vi "Camera_Config_Specific_Attributes_2.0.vi"(4 "Crop?":bool, 5 "Camera":T5, 6 "Detect Movement":bool, 8 "error in (no error)":errorcluster, 10 "Refnum in":T2, 11 "Data":T1={"Camera 1"={"Camera1"="", "Cam 1"=FALSE, "CAM1 Model"=enum."a2A5328-15ucBAS", "Cam1 ID"=0}, "Camera 2"={"Camera2"="", "Cam 2"=FALSE, "CAM2 Model"=enum."a2A5328-15ucBAS", "Cam2 ID"=0}, "Image"={"Camera1_Img"=refnum, "Camera2_Img"=refnum, "Img1_Orig_Disp"=refnum, "Img2_Orig_Disp"=refnum, "Img1_Orig_RGB"=refnum, "Img2_Orig_RGB"=refnum, "Blue_Plane_Extract"=refnum, "Subtracted_Plane"=refnum, "Img1_Binary"=refnum, "Img2_Binary"=refnum, "Crop_Mask"=refnum, "Img1_Save"=refnum, "Img2_Save"=refnum, "Img1_Cali_Full"=refnum, "Img2_Cali_Full"=refnum, "Img1_Cali_Detect"=refnum, "Img2_Cali_Detect"=refnum}, "Ques"={"Cam 1 queue"=refnum, "Cam 2 queue"=refnum, "Cam 1 - save queue"=refnum, "Cam 2 - save queue"=refnum, "Image Process Queue Size"=500, "Image Save Queue Size"=500, "Overload threshold"=500, "Max large object threshold"=0}, "Arduino SRS"={"Pinch-valve"="", "Actuator"=FALSE, "Arduino Uno"="", "Valve state"=enum."Open"}, "Pump"={"Port"="", "Connection"=FALSE, "Flush Size"=0, "Command"="", "Pump Size"=enum."None", "Pump"="", "Ready"=FALSE}, "Camera settings"={"Detection settings"={"Sample size threshold"=500, "Detection Region %"=30.0, "Timeout Sample"=200}, "Lens/camera settings"={"Aperture"=enum."Item 0", "Legacy Cam Attributes"=FALSE, "Max Framerate"=100, "Exposure Time"=1000.0, "Framerate"=15}, "Crop settings"={"Cam1"={"Rectangle 1"={"Left"=0, "Top"=0, "Right"=0, "Bottom"=0, "Rotation"=0.0}, "Camera Orientation 1"="", "Pixel to mm 1"=0.0}, "Cam2"={"Rectangle 2"={"Left"=0, "Top"=0, "Right"=0, "Bottom"=0, "Rotation"=0.0}, "Camera Orientation 2"="", "Pixel to mm 2"=0.0}}}, "Arduino ISS"={"Mega F3"="", "Phase3"=FALSE, "Barcode"="", "Sorting sys."=FALSE, "Initial size"=0.0, "Size Interval"=0.0, "Mun. of containers"=0.0, "Container nr."=0.0, "Arduino Mega"=""}, "Img_Capt"=FALSE, "Empty_Refill"=FALSE, "I don't think is in use"={"Light intensity"=100}, "Extended setup"={"Location"="Station", "Latitude"="Station", "Longitude"="Station", "Determiner"="Station", "Sex"="Station", "Station"="", "Collection date"=""}, "Main interface"={"Sample Name"="Test Sample", "Operator"="JFR", "Species Name"="", "Other Notes"=""}, "Tap1"=0, "SystemVersion"=0, "System Serial"="", "Exit"=FALSE, "Kuvette Full"=FALSE, "Core JKI"={"Current VI Reference"=refnum, "Close Panel on Exit?"=FALSE}, "Calibration"={"Calibration 1"=path "C:/Users/au540322/Desktop/IHS_Project/images/Debris/Debris_0/Debris_0_2019_06_01-23-32-49-686.PNG", "Calibration 2"=path "C:/Users/au540322/Desktop/IHS_Project/images/Debris/Debris_0/Debris_0_2019_06_01-23-32-49-686.PNG", "Detect 1"=path "C:/Users/au540322/Desktop/IHS_Project/images/Debris/Debris_0/Debris_0_2019_06_01-23-32-49-686.PNG", "Detect 2"=path "C:/Users/au540322/Desktop/IHS_Project/images/Debris/Debris_0/Debris_0_2019_06_01-23-32-49-686.PNG"}, "Auto Flush"=FALSE, "Status History"="", "Timestamp Start"=""} {"SystemVersion" items=["Standard", "XL"]; "Tap1" items=["Session Data", "Extended Setup", "Buffer", "Camera", "Dispenser", "Stats", "Connections"]; "I don't think is in use"."Light intensity" scale=0.0..100.0; "Camera settings"."Crop settings"."Cam2"."Rectangle 2"."Rotation" format="%.2f"; "Camera settings"."Crop settings"."Cam2"."Rectangle 2"."Left" scale=0.0..1024.0; "Camera settings"."Crop settings"."Cam2"."Rectangle 2"."Right" scale=0.0..1024.0; "Camera settings"."Crop settings"."Cam1"."Rectangle 1"."Rotation" format="%.2f"; "Camera settings"."Crop settings"."Cam1"."Rectangle 1"."Left" scale=0.0..1024.0; "Camera settings"."Crop settings"."Cam1"."Rectangle 1"."Right" scale=0.0..1024.0; "Camera settings"."Lens/camera settings"."Framerate" min=1; "Camera settings"."Lens/camera settings"."Max Framerate" min=1; "Camera settings"."Detection settings"."Sample size threshold" min=1; "Pump"."Flush Size" min=0 max=6000 step=100; "Ques"."Overload threshold" min=1; "Ques"."Image Save Queue Size" min=1; "Ques"."Image Process Queue Size" min=1}) -> (0 "error out":errorcluster, 3 "Refnum out":T2)   [LabVIEW 2024]
uses:
  <vilib>/userDefined/High Color/IMAQdx.ctl
  Camera_ID.ctl
  controls/Data_JKI.ctl
  <vilib>/vision/Image Controls.llb/IMAQ Image.ctl
  <resource>/objmgr/imaqdx.rc
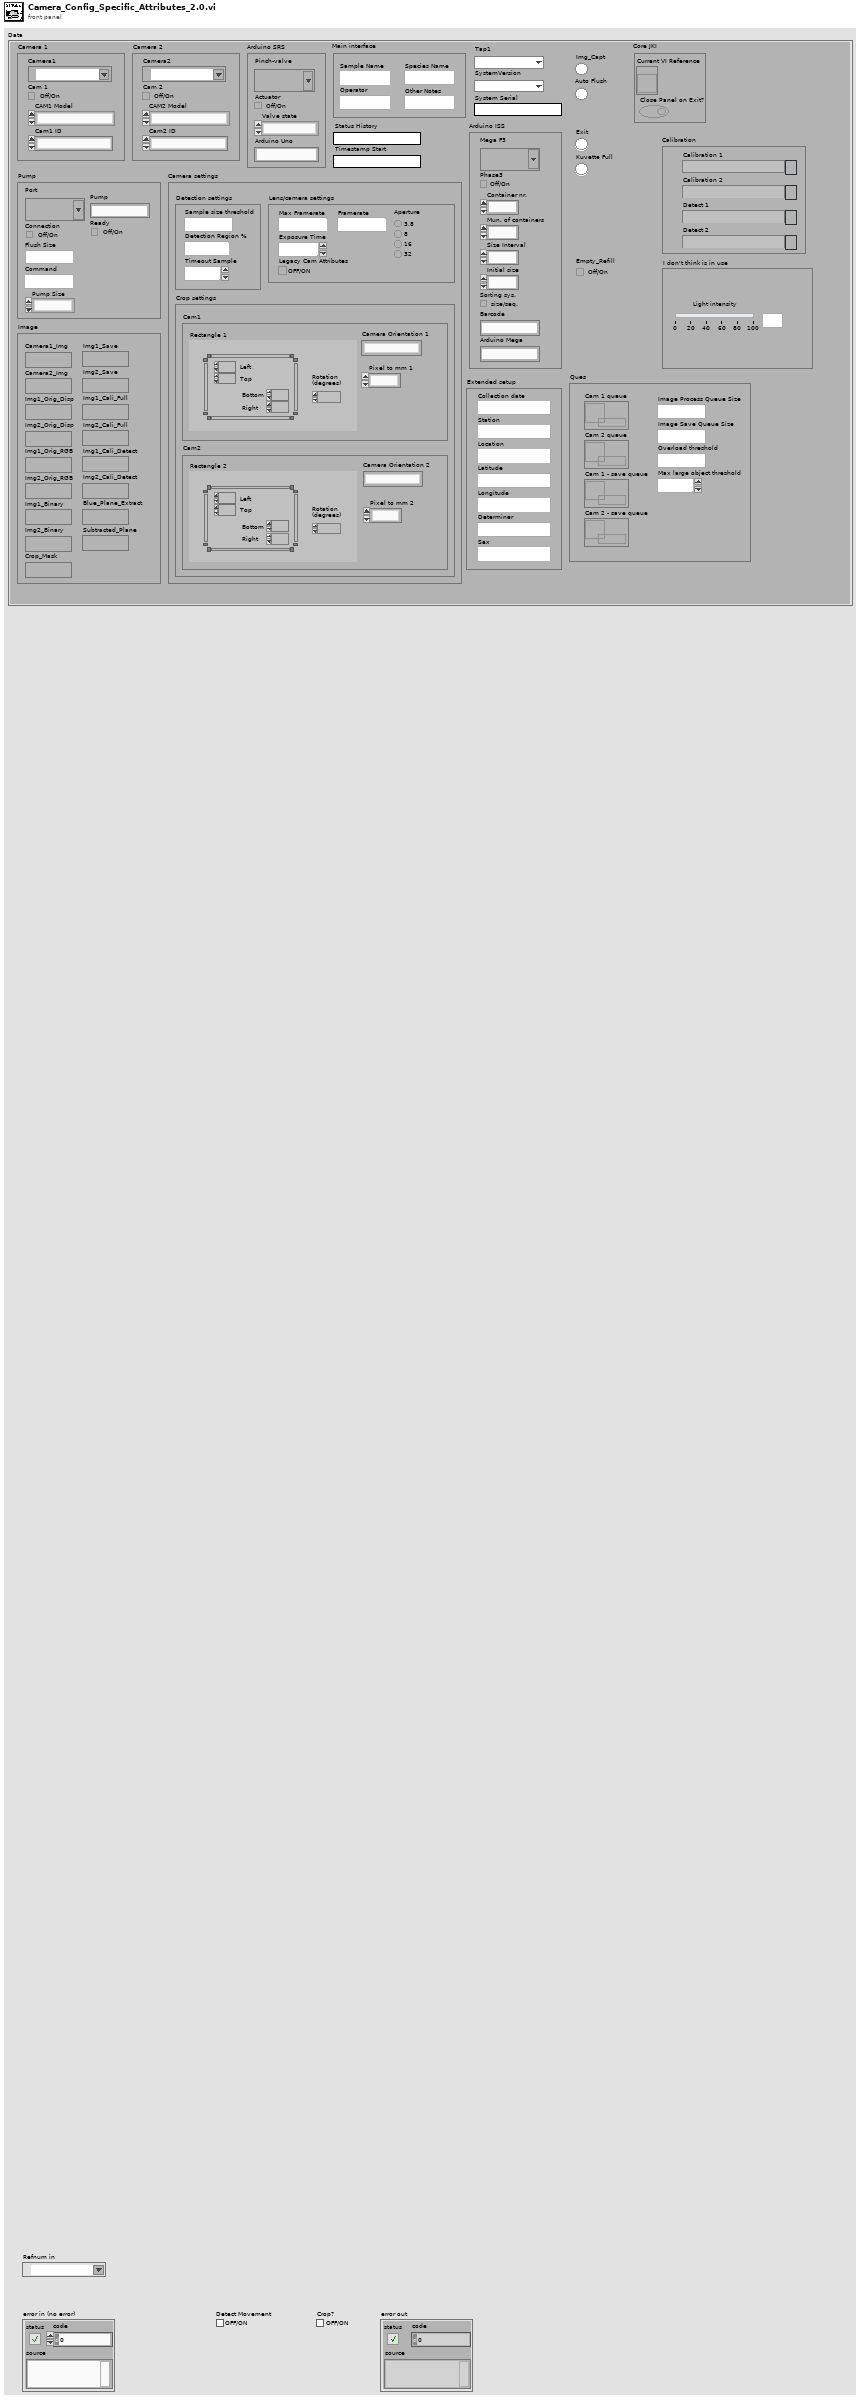
[diagram p1: front panel]
types:
  T1 = typedef "Data_JKI.ctl" = cluster{"Camera 1":cluster{"Camera1":T2, "Cam 1":bool, "CAM1 Model":enum16{"a2A5328-15ucBAS", "acA1920-155uc"}, "Cam1 ID":i32}, "Camera 2":cluster{"Camera2":T2, "Cam 2":bool, "CAM2 Model":enum16{"a2A5328-15ucBAS", "acA1920-155uc"}, "Cam2 ID":i32}, "Image":cluster{"Camera1_Img":T3, "Camera2_Img":T3, "Img1_Orig_Disp":T3, "Img2_Orig_Disp":T3, "Img1_Orig_RGB":T3, "Img2_Orig_RGB":T3, "Blue_Plane_Extract":T3, "Subtracted_Plane":T3, "Img1_Binary":T3, "Img2_Binary":T3, "Crop_Mask":T3, "Img1_Save":T3, "Img2_Save":T3, "Img1_Cali_Full":T3, "Img2_Cali_Full":T3, "Img1_Cali_Detect":T3, "Img2_Cali_Detect":T3}, "Ques":cluster{"Cam 1 queue":refnum<queue>, "Cam 2 queue":refnum<queue>, "Cam 1 - save queue":refnum<queue>, "Cam 2 - save queue":refnum<queue>, "Image Process Queue Size":i32, "Image Save Queue Size":i32, "Overload threshold":i32, "Max large object threshold":i32}, "Arduino SRS":cluster{"Pinch-valve":refnum<visa-resource-name>, "Actuator":bool, "Arduino Uno":string, "Valve state":enum16{"Standby", "Close", "Open"}}, "Pump":cluster{"Port":refnum<visa-resource-name>, "Connection":bool, "Flush Size":i32, "Command":string, "Pump Size":enum16{"None", "Small", "Large"}, "Pump":string, "Ready":bool}, "Camera settings":cluster{"Detection settings":cluster{"Sample size threshold":i32, "Detection Region %":dbl, "Timeout Sample":i32}, "Lens/camera settings":cluster{"Aperture":enum32{"Item 0", "Item 1", "Item 2", "Item 3"}, "Legacy Cam Attributes":bool, "Max Framerate":i32, "Exposure Time":dbl, "Framerate":i32}, "Crop settings":cluster{"Cam1":cluster{"Rectangle 1":T4, "Camera Orientation 1":string, "Pixel to mm 1":dbl}, "Cam2":cluster{"Rectangle 2":T4, "Camera Orientation 2":string, "Pixel to mm 2":dbl}}}, "Arduino ISS":cluster{"Mega F3":refnum<visa-resource-name>, "Phase3":bool, "Barcode":string, "Sorting sys.":bool, "Initial size":dbl, "Size Interval":dbl, "Mun. of containers":dbl, "Container nr.":dbl, "Arduino Mega":string}, "Img_Capt":bool, "Empty_Refill":bool, "I don't think is in use":cluster{"Light intensity":i32}, "Extended setup":cluster{"Location":string, "Latitude":string, "Longitude":string, "Determiner":string, "Sex":string, "Station":string, "Collection date":string}, "Main interface":cluster{"Sample Name":string, "Operator":string, "Species Name":string, "Other Notes":string}, "Tap1":u16, "SystemVersion":u16, "System Serial":string, "Exit":bool, "Kuvette Full":bool, "Core JKI":cluster{"Current VI Reference":refnum<vi>, "Close Panel on Exit?":bool}, "Calibration":cluster{"Calibration 1":path, "Calibration 2":path, "Detect 1":path, "Detect 2":path}, "Auto Flush":bool, "Status History":string, "Timestamp Start":string}
  T2 = typedef "IMAQdx.ctl" = refnum<k21>
  T3 = typedef "IMAQ Image.ctl" = refnum<image>
  T4 = typedef "IMAQ Rectangle" = cluster{"Left":i32, "Top":i32, "Right":i32, "Bottom":i32, "Rotation":dbl}
  T5 = typedef "Camera_ID.ctl" = enum16{"Camera 1", "Camera 2"}
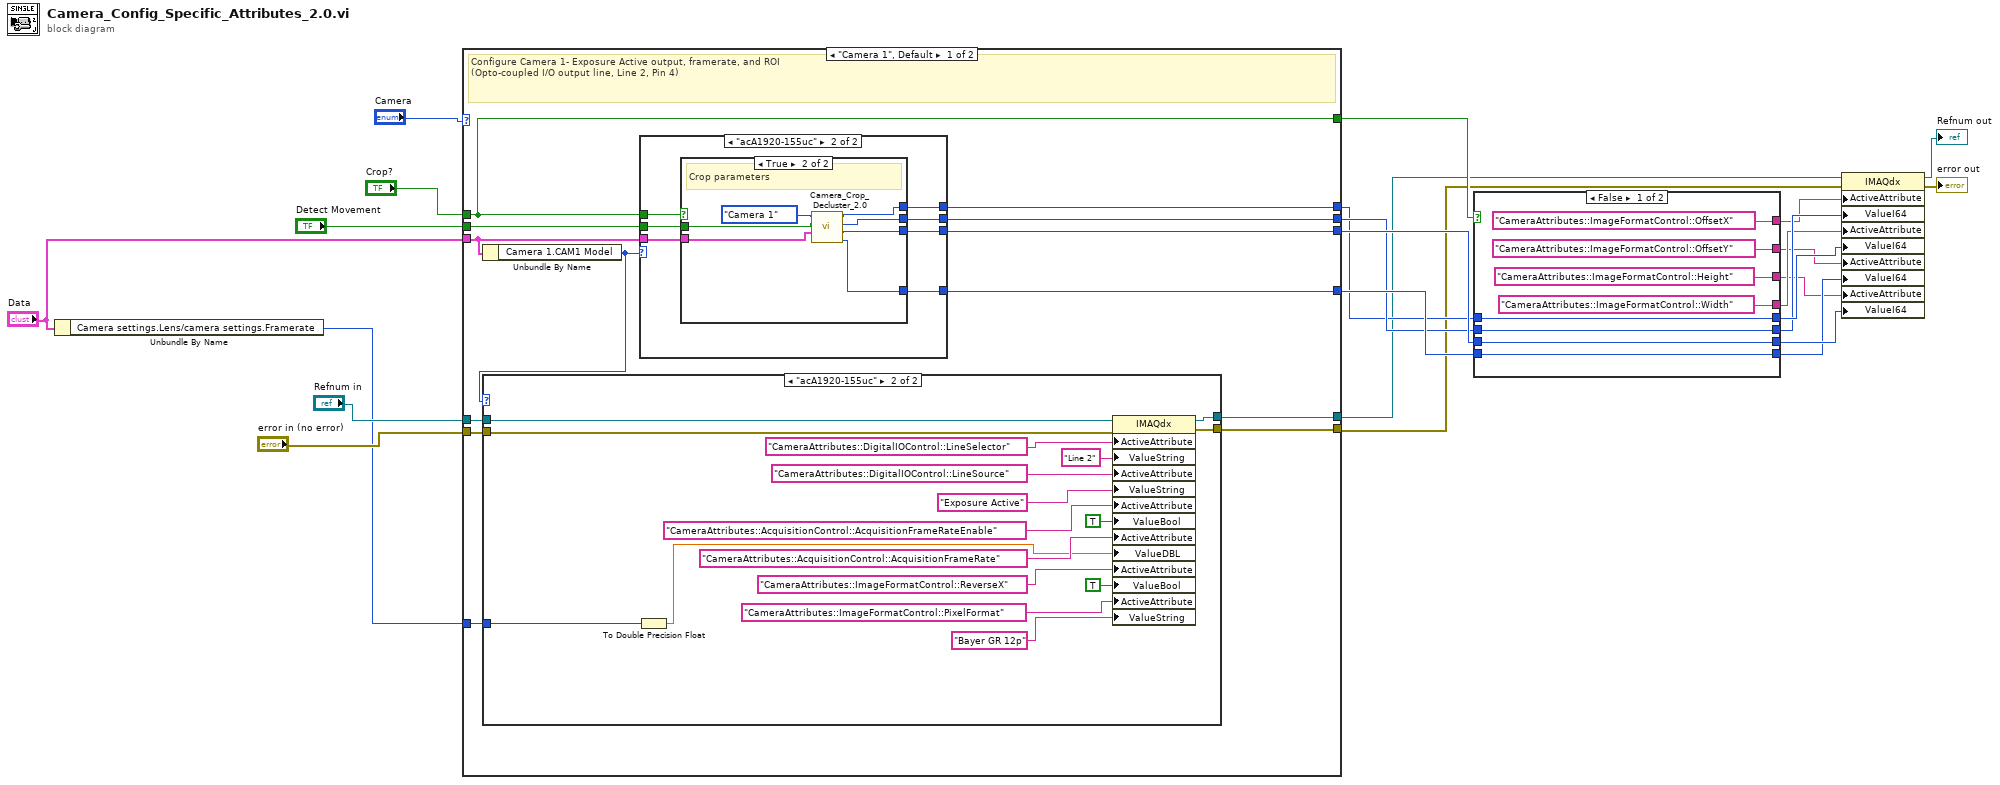
[diagram p0: block diagram]
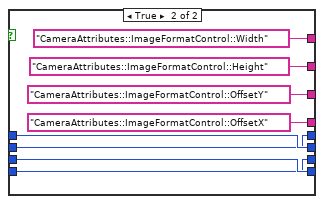
[diagram p2: hidden frame]
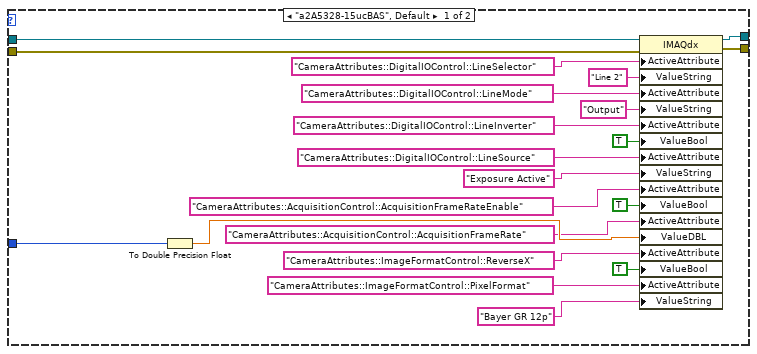
[diagram p3: hidden frame]
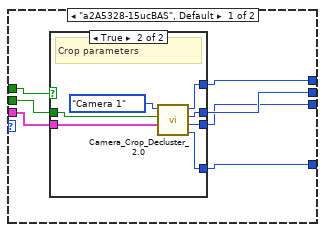
[diagram p4: hidden frame]
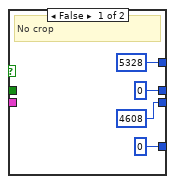
[diagram p5: hidden frame]
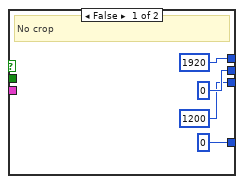
[diagram p6: hidden frame]
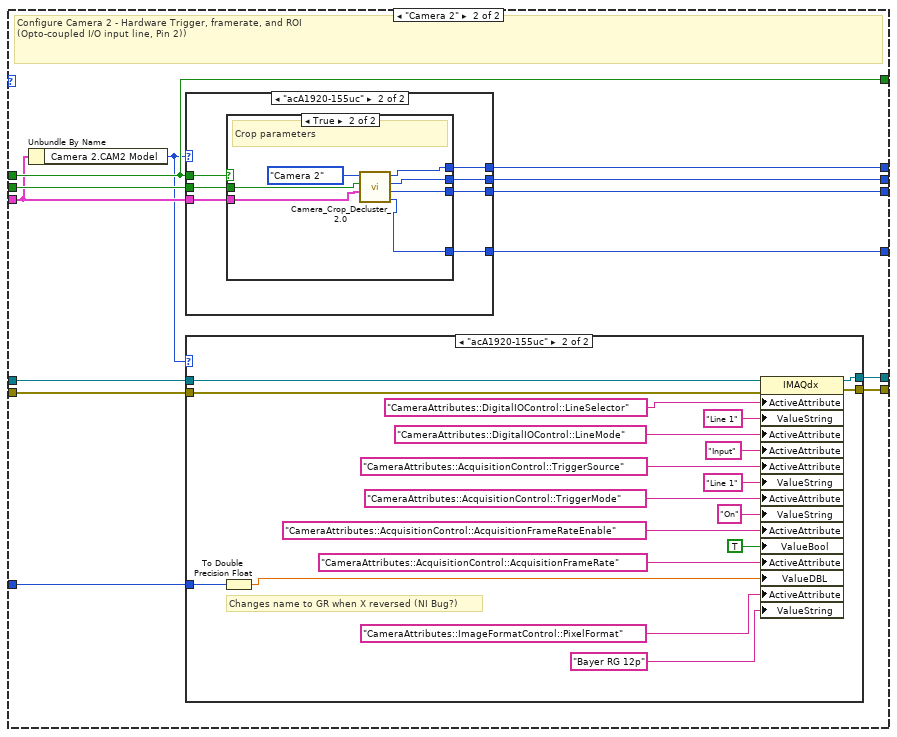
[diagram p7: hidden frame]
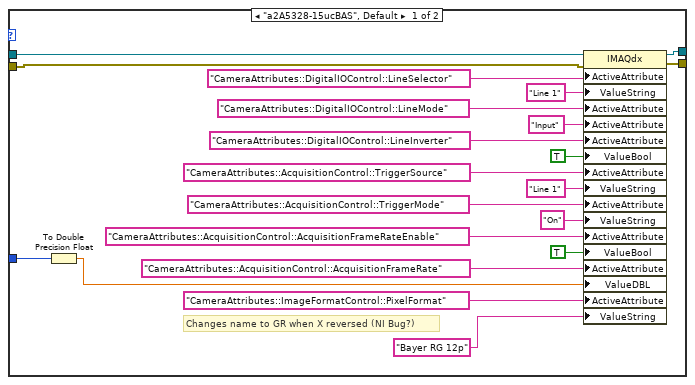
[diagram p8: hidden frame]
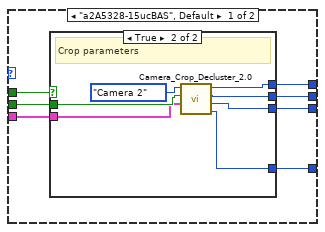
[diagram p9: hidden frame]
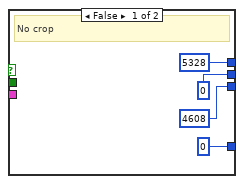
[diagram p10: hidden frame]
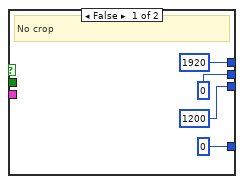
[diagram p11: hidden frame]
diagram:
  n1 = Unbundle By Name("Data") -> ("Camera settings.Lens/camera settings.Framerate"=w4:i32)
  n2 = case shown="\"Camera 1\", Default" "Camera" {
    tunnel: "Refnum in" -> [w37 w118]
    tunnel: [w36 w117] -> w2
    tunnel: [w35 w116] -> w1
    tunnel: w4 -> [w27 w113]
    tunnel: [w33 w124] -> w17
    tunnel: [w34 w123] -> w14
    tunnel: [w31 w121] -> w19
    tunnel: [w32 w122] -> w15
    tunnel: "Crop?" -> [w30 w120]
    tunnel: [w30 w120] -> w12
    tunnel: "Data" -> [w26 w114]
    tunnel: "Detect Movement" -> [w29 w119]
    tunnel: "error in (no error)" -> [w28 w115]
    frame "Camera 1", Default {
      # "Configure Camera 1- Exposure Active output, framerate, and ROI\n(Opto-coupled I/O output line, Line 2, Pin 4)"
      n3 = Unbundle By Name(w26) -> ("Camera 1.CAM1 Model"=w25:enum16{"a2A5328-15ucBAS", "acA1920-155uc"})
      n4 = case shown="\"acA1920-155uc\"" w25 {
        tunnel: w37 -> [w58 w75]
        tunnel: [w56 w74] -> w36
        tunnel: [w55 w73] -> w35
        tunnel: w28 -> [w57 w71]
        tunnel: w27 -> [w44 w60]
        frame "a2A5328-15ucBAS", Default {
          n5 = To Double Precision Float(number=w44) -> (double precision float=w43:dbl)
          n6 = property class="IMAQdx"(reference=w58, error in=w57, "ActiveAttribute"="CameraAttributes::DigitalIOControl::LineSelector", "ValueString"="Line 2", "ActiveAttribute"="CameraAttributes::DigitalIOControl::LineMode", "ValueString"="Output", "ActiveAttribute"="CameraAttributes::DigitalIOControl::LineInverter", "ValueBool"=TRUE, "ActiveAttribute"="CameraAttributes::DigitalIOControl::LineSource", "ValueString"="Exposure Active", "ActiveAttribute"="CameraAttributes::AcquisitionControl::AcquisitionFrameRateEnable", "ValueBool"=TRUE, "ActiveAttribute"="CameraAttributes::AcquisitionControl::AcquisitionFrameRate", "ValueDBL"=w43, "ActiveAttribute"="CameraAttributes::ImageFormatControl::ReverseX", "ValueBool"=TRUE, "ActiveAttribute"="CameraAttributes::ImageFormatControl::PixelFormat", "ValueString"="Bayer GR 12p") -> (reference out=w56:T2, error out=w55:errorcluster)
        }
        frame "acA1920-155uc" {
          n7 = To Double Precision Float(number=w60) -> (double precision float=w59:dbl)
          n8 = property class="IMAQdx"(reference=w75, error in=w71, "ActiveAttribute"="CameraAttributes::DigitalIOControl::LineSelector", "ValueString"="Line 2", "ActiveAttribute"="CameraAttributes::DigitalIOControl::LineSource", "ValueString"="Exposure Active", "ActiveAttribute"="CameraAttributes::AcquisitionControl::AcquisitionFrameRateEnable", "ValueBool"=TRUE, "ActiveAttribute"="CameraAttributes::AcquisitionControl::AcquisitionFrameRate", "ValueDBL"=w59, "ActiveAttribute"="CameraAttributes::ImageFormatControl::ReverseX", "ValueBool"=TRUE, "ActiveAttribute"="CameraAttributes::ImageFormatControl::PixelFormat", "ValueString"="Bayer GR 12p") -> (reference out=w74:T2, error out=w73:errorcluster)
        }
      }
      n9 = case shown="\"acA1920-155uc\"" w25 {
        tunnel: [w79 w100] -> w34
        tunnel: [w77 w99] -> w33
        tunnel: [w78 w98] -> w32
        tunnel: [w76 w97] -> w31
        tunnel: w30 -> [w82 w96]
        tunnel: w26 -> [w80 w95]
        tunnel: w29 -> [w81 w94]
        frame "a2A5328-15ucBAS", Default {
          n10 = case shown="True" w82 {
            tunnel: [5328 w90] -> w79
            tunnel: [4608 w88] -> w77
            tunnel: [i64 0 w89] -> w78
            tunnel: [0 w87] -> w76
            tunnel: w80 -> [_ w91]
            tunnel: w81 -> [_ w92]
            frame False {
              # "No crop"
            }
            frame True {
              # "Crop parameters"
              n11 = call "Camera_Crop_Decluster_2.0.vi"("Data"=w91, "Detect Movement"=w92, "Camera"=Camera_ID."Camera 1") -> ("OffsetY"=w87:i64, "Height"=w88:i64, "OffsetX"=w89:i64, "Width"=w90:i64)  [unwired: 5 in]
            }
          }
        }
        frame "acA1920-155uc" {
          n12 = case shown="True" w96 {
            tunnel: [i64 1920 w108] -> w100
            tunnel: [1200 w106] -> w99
            tunnel: [i64 0 w107] -> w98
            tunnel: [0 w105] -> w97
            tunnel: w95 -> [_ w109]
            tunnel: w94 -> [_ w110]
            frame False {
              # "No crop"
            }
            frame True {
              # "Crop parameters"
              n13 = call "Camera_Crop_Decluster_2.0.vi"("Data"=w109, "Detect Movement"=w110, "Camera"=Camera_ID."Camera 1") -> ("OffsetY"=w105:i64, "Height"=w106:i64, "OffsetX"=w107:i64, "Width"=w108:i64)  [unwired: 5 in]
            }
          }
        }
      }
    }
    frame "Camera 2" {
      # "Configure Camera 2 - Hardware Trigger, framerate, and ROI \n(Opto-coupled I/O input line, Pin 2))"
      n14 = Unbundle By Name(w114) -> ("Camera 2.CAM2 Model"=w112:enum16{"a2A5328-15ucBAS", "acA1920-155uc"})
      n15 = case shown="\"acA1920-155uc\"" w112 {
        tunnel: [w166 w189] -> w124
        tunnel: [w168 w188] -> w123
        tunnel: [w167 w187] -> w122
        tunnel: [w165 w186] -> w121
        tunnel: w120 -> [w171 w185]
        tunnel: w114 -> [w170 w184]
        tunnel: w119 -> [w169 w183]
        frame "a2A5328-15ucBAS", Default {
          n16 = case shown="True" w171 {
            tunnel: [i64 4608 w177] -> w166
            tunnel: [i64 5328 w179] -> w168
            tunnel: [i64 0 w178] -> w167
            tunnel: [i64 0 w176] -> w165
            tunnel: w170 -> [_ w180]
            tunnel: w169 -> [_ w181]
            frame False {
              # "No crop"
            }
            frame True {
              # "Crop parameters"
              n17 = call "Camera_Crop_Decluster_2.0.vi"("Data"=w180, "Detect Movement"=w181, "Camera"=Camera_ID."Camera 2") -> ("OffsetY"=w176:i64, "Height"=w177:i64, "OffsetX"=w178:i64, "Width"=w179:i64)  [unwired: 5 in]
            }
          }
        }
        frame "acA1920-155uc" {
          n18 = case shown="True" w185 {
            tunnel: [i64 1200 w195] -> w189
            tunnel: [i64 1920 w197] -> w188
            tunnel: [i64 0 w196] -> w187
            tunnel: [i64 0 w194] -> w186
            tunnel: w184 -> [_ w198]
            tunnel: w183 -> [_ w199]
            frame False {
              # "No crop"
            }
            frame True {
              # "Crop parameters"
              n19 = call "Camera_Crop_Decluster_2.0.vi"("Data"=w198, "Detect Movement"=w199, "Camera"=Camera_ID."Camera 2") -> ("OffsetY"=w194:i64, "Height"=w195:i64, "OffsetX"=w196:i64, "Width"=w197:i64)  [unwired: 5 in]
            }
          }
        }
      }
      n20 = case shown="\"acA1920-155uc\"" w112 {
        tunnel: w118 -> [w129 w163]
        tunnel: [w131 w162] -> w117
        tunnel: [w130 w161] -> w116
        tunnel: w115 -> [w128 w160]
        tunnel: w113 -> [w125 w155]
        frame "a2A5328-15ucBAS", Default {
          # "Changes name to GR when X reversed (NI Bug?)"
          n21 = To Double Precision Float(number=w125) -> (double precision float=w140:dbl)
          n22 = property class="IMAQdx"(reference=w129, error in=w128, "ActiveAttribute"="CameraAttributes::DigitalIOControl::LineSelector", "ValueString"="Line 1", "ActiveAttribute"="CameraAttributes::DigitalIOControl::LineMode", "ActiveAttribute"="Input", "ActiveAttribute"="CameraAttributes::DigitalIOControl::LineInverter", "ValueBool"=TRUE, "ActiveAttribute"="CameraAttributes::AcquisitionControl::TriggerSource", "ValueString"="Line 1", "ActiveAttribute"="CameraAttributes::AcquisitionControl::TriggerMode", "ValueString"="On", "ActiveAttribute"="CameraAttributes::AcquisitionControl::AcquisitionFrameRateEnable", "ValueBool"=TRUE, "ActiveAttribute"="CameraAttributes::AcquisitionControl::AcquisitionFrameRate", "ValueDBL"=w140, "ActiveAttribute"="CameraAttributes::ImageFormatControl::PixelFormat", "ValueString"="Bayer RG 12p") -> (reference out=w131:T2, error out=w130:errorcluster)
        }
        frame "acA1920-155uc" {
          # "Changes name to GR when X reversed (NI Bug?)"
          n23 = To Double Precision Float(number=w155) -> (double precision float=w154:dbl)
          n24 = property class="IMAQdx"(reference=w163, error in=w160, "ActiveAttribute"="CameraAttributes::DigitalIOControl::LineSelector", "ValueString"="Line 1", "ActiveAttribute"="CameraAttributes::DigitalIOControl::LineMode", "ActiveAttribute"="Input", "ActiveAttribute"="CameraAttributes::AcquisitionControl::TriggerSource", "ValueString"="Line 1", "ActiveAttribute"="CameraAttributes::AcquisitionControl::TriggerMode", "ValueString"="On", "ActiveAttribute"="CameraAttributes::AcquisitionControl::AcquisitionFrameRateEnable", "ValueBool"=TRUE, "ActiveAttribute"="CameraAttributes::AcquisitionControl::AcquisitionFrameRate", "ValueDBL"=w154, "ActiveAttribute"="CameraAttributes::ImageFormatControl::PixelFormat", "ValueString"="Bayer RG 12p") -> (reference out=w162:T2, error out=w161:errorcluster)
        }
      }
    }
  }
  n25 = case shown="False" w12 {
    tunnel: ["CameraAttributes::ImageFormatControl::Height" ("ActiveAttribute") "CameraAttributes::ImageFormatControl::OffsetY" ("ActiveAttribute")] -> w6
    tunnel: ["CameraAttributes::ImageFormatControl::OffsetY" ("ActiveAttribute") "CameraAttributes::ImageFormatControl::Height" ("ActiveAttribute")] -> w7
    tunnel: ["CameraAttributes::ImageFormatControl::Width" ("ActiveAttribute") "CameraAttributes::ImageFormatControl::OffsetX" ("ActiveAttribute")] -> w8
    tunnel: ["CameraAttributes::ImageFormatControl::OffsetX" ("ActiveAttribute") "CameraAttributes::ImageFormatControl::Width" ("ActiveAttribute")] -> w9
    tunnel: [w203 w212] -> w13
    tunnel: w14 -> [w204 w212]
    tunnel: w15 -> [w203 w211]
    tunnel: [w204 w211] -> w16
    tunnel: w17 -> [w202 w210]
    tunnel: [w201 w210] -> w18
    tunnel: w19 -> [w201 w209]
    tunnel: [w202 w209] -> w20
    frame False {
    }
    frame True {
    }
  }
  n26 = property class="IMAQdx"(reference=w2, error in=w1, "ActiveAttribute"=w9, "ValueI64"=w13, "ActiveAttribute"=w8, "ValueI64"=w16, "ActiveAttribute"=w7, "ValueI64"=w18, "ActiveAttribute"=w6, "ValueI64"=w20) -> (reference out=→"Refnum out":T2, error out=→"error out":errorcluster)
